vi "Ramp Example.vi"() -> ()   [LabVIEW 2010]
uses:
  <vilib>/addons/control/pid/pid.llb/PID Output Rate Limiter (DBL).vi
  <vilib>/ptbypt/NI_PtbyPt.lvlib
  <vilib>/addons/control/pid/NI_PID_pid.lvlib
panel:
  in  "output rate (EGU/min)":dbl=200.0
  in  "Average Filter Sample Length":i32=10
  in  "Low Pass Filter Average Length":dbl=0.05
  in  "Joystick Input":dbl(slide) scale=-1.0..1.0
  out "Input to Motor":T1(graph)
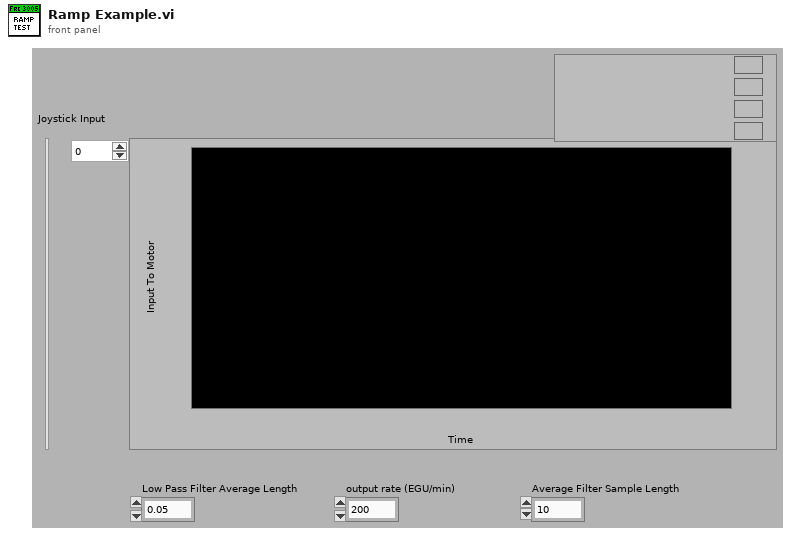
[diagram p1: front panel]
types:
  T1 = cluster{"Joystick Input":dbl, "upper limit":dbl, "upper limit":dbl, "output":dbl}
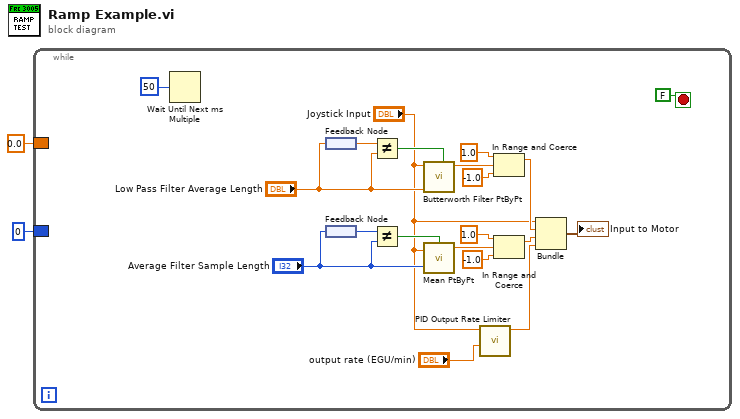
[diagram p0: block diagram]
diagram:
  n1 = while {
    border: 0 ("Average Filter Sample Length") -> [_]
    border: 0.0 ("Low Pass Filter Average Length") -> [_]
    stop <- FALSE stop-if-true
    n2 = Wait Until Next ms Multiple(millisecond multiple=u32 50) -> ()  [unwired: 1 out]
    n3 = feedback #1() -> (w8:dbl)
    n4 = feedback-in #1("Low Pass Filter Average Length") -> ()
    n5 = feedback-in #2("Average Filter Sample Length") -> ()
    n6 = feedback #2() -> (w11:i32)
    n7 = Not Equal?(x=w8, y="Low Pass Filter Average Length") -> (x != y?=w6:bool)
    n8 = Not Equal?(x=w11, y="Average Filter Sample Length") -> (x != y?=w9:bool)
    n9 = call <vilib>:"Butterworth Filter PtByPt.vi"("initialize"=w6, "low cutoff freq: fl"="Low Pass Filter Average Length", "x"="Joystick Input") -> ("Filtered x"=w19:dbl)  [unwired: 6 in, 1 out]
    n10 = call <vilib>:"Mean PtByPt.vi"("x"="Joystick Input", "sample length"="Average Filter Sample Length", "initialize"=w9) -> ("mean"=w13:dbl)  [unwired: 1 in, 1 out]
    n11 = call-poly <vilib>:"PID Output Rate Limiter.vi"("output rate (EGU/min)"="output rate (EGU/min)", "input (controller output)"="Joystick Input") -> ("output"=w3:dbl)  [unwired: 6 in, 1 out]
    n12 = In Range and Coerce(upper limit=1.0, x=w19, lower limit=-1.0) -> (coerced(x)=w18:dbl)  [unwired: 1 out]
    n13 = In Range and Coerce(upper limit=1.0, x=w13, lower limit=-1.0) -> (coerced(x)=w12:dbl)  [unwired: 1 out]
    n14 = Bundle("Joystick Input"="Joystick Input", "upper limit"=w18, "upper limit"=w12, "output"=w3) -> (→"Input to Motor":T1)  [unwired: 1 in]
  }
